vi "Display event.vi"(4 "No hit color":T1, 6 "Hit color":T1, 8 "error in (no error)":errorcluster, 10 "Hits to display":T3, 11 "Event Display in":refnum<vi>) -> (0 "error out":errorcluster, 3 "Event Display out":refnum<vi>)   [LabVIEW 2016]
uses:
  Typedefs/Coincidence.ctl
  <vilib>/Utility/miscctls.llb/LVRGBAColorTypeDef.ctl
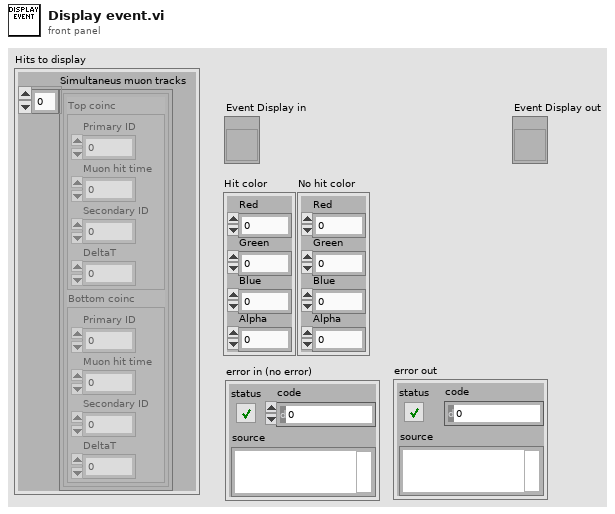
[diagram p1: front panel]
types:
  T1 = typedef "LVRGBAColorTypeDef.ctl" = cluster{"Red":sgl, "Green":sgl, "Blue":sgl, "Alpha":sgl}
  T2 = typedef "Coincidence.ctl" = cluster{"Primary ID":i8, "Muon hit time":u64, "Secondary ID":i8, "DeltaT":i32}
  T3 = cluster{"Simultaneus muon tracks":cluster{"Top coinc":T2, "Bottom coinc":T2}[]}
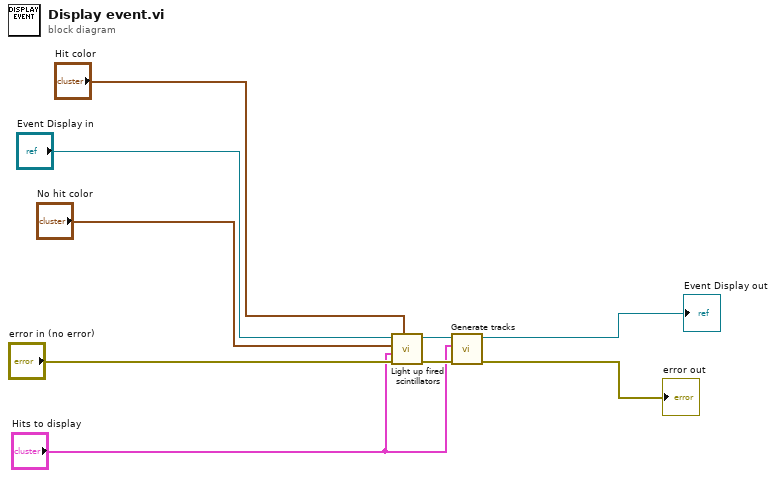
[diagram p0: block diagram]
diagram:
  n1 = call "Light up fired scintillators.vi"("Hit color"="Hit color", "error in (no error)"="error in (no error)", "Hits to display"="Hits to display", "No hit color"="No hit color", "SceneObject in"="Event Display in") -> ("error out"=w5:errorcluster, "SceneObject out"=w3:refnum<vi>)  [unwired: 5 in]
  n2 = call "Generate tracks.vi"("error in (no error)"=w5, "Hits to display"="Hits to display", "Event display in"=w3) -> ("error out"=→"error out":errorcluster, "Event display out"=→"Event Display out":refnum<vi>)  [unwired: 7 in]
